vi "GetInfo.vi"() -> (3 "concatenated string":string)   [LabVIEW 2024]
uses:
  global.vi
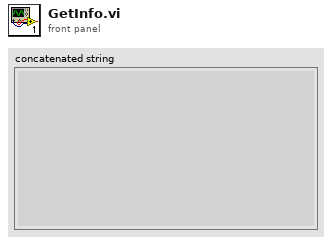
[diagram p1: front panel]
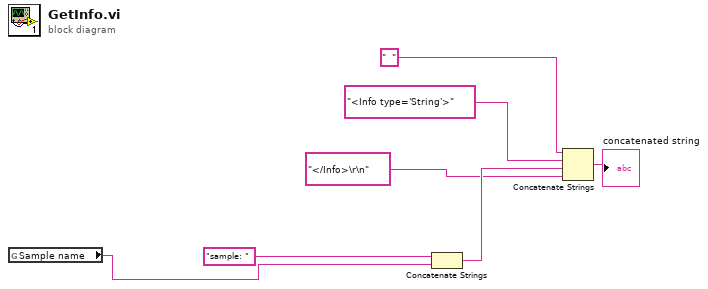
[diagram p0: block diagram]
diagram:
  n1 = global read "global.vi" "Sample name"() -> (w6:string)
  n2 = Concatenate Strings("sample: " ("string"), w6) -> (w5:string)
  n3 = Concatenate Strings("  ", "<Info type='String'>" ("string"), w5, "</Info>\r\n" ("string")) -> (→"concatenated string":string)
